vi "Camera Begin.vi"() -> ()   [LabVIEW 2013]
uses:
  <vilib>/Rock Robotics/WPI/Camera/WPI_CameraWhite Balance Values.ctl
  <vilib>/Rock Robotics/WPI/Camera/WPI_CameraFrameRate.ctl
  <vilib>/Rock Robotics/WPI/Camera/WPI_CameraExposure Values.ctl
  <vilib>/Rock Robotics/WPI/Camera/WPI_CameraImageSize.ctl
  <vilib>/Rock Robotics/SystemInterfaces/AI/FPGA_AIChannel.ctl
  <vilib>/Rock Robotics/SystemInterfaces/Typedef/FPGA_TypedefAnalogModule.ctl
panel:
  in  "Camera 2":T5={"Camera Address"="192.168.0.90", "Compression"=0, "White Balance"=enum."Auto", "Frame Rate (fps)"=30, "Exposure"=enum."Auto", "Image Size"=enum."320x240", "Brightness"=50, "refnum name"="My Camera RefNum"} {"Brightness" min=0 max=100; "Frame Rate (fps)" min=1 max=30; "Compression" min=0 max=100}
  in  "Camera 1":T5={"Camera Address"="192.168.0.90", "Compression"=0, "White Balance"=enum."Auto", "Frame Rate (fps)"=30, "Exposure"=enum."Auto", "Image Size"=enum."320x240", "Brightness"=50, "refnum name"="My Camera RefNum"} {"Brightness" min=0 max=100; "Frame Rate (fps)" min=1 max=30; "Compression" min=0 max=100}
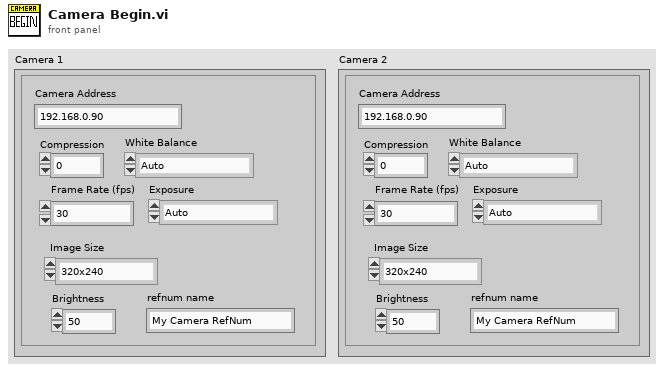
[diagram p1: front panel]
types:
  T1 = typedef "WPI_CameraWhite Balance Values.ctl" = enum16{"Auto", "Fixed indoor", "Fixed outdoor 1", "Fixed outdoor 2", "Fixed fluorescent 1", "Fixed fluorescent 2", "Hold current"}
  T2 = typedef "WPI_CameraFrameRate.ctl" = u32
  T3 = typedef "WPI_CameraExposure Values.ctl" = enum16{"Auto", "Flicker-free 50 Hz", "Flicker-free 60 Hz", "Hold current"}
  T4 = typedef "WPI_CameraImageSize.ctl" = enum16{"640x480", "320x240", "160x120"}
  T5 = cluster{"Camera Address":string, "Compression":i32, "White Balance":T1, "Frame Rate (fps)":T2, "Exposure":T3, "Image Size":T4, "Brightness":i32, "refnum name":string}
  T6 = typedef "FPGA_TypedefAnalogModule.ctl" = enum16{"Analog Module 1", "Analog Module 2"}
  T7 = typedef "FPGA_AIChannel.ctl" = enum8{"AI 1", "AI 2", "AI 3", "AI 4", "AI 5", "AI 6", "AI 7", "AI 8", "Invalid"}
  T8 = typedef "WPI_AnalogChannelDevRef.ctl" = cluster{"DevStatus":errorcluster, "Analog Module":T6, "Analog Channel":T7}
  T9 = typedef "WPI_CameraDevRef.ctl" = cluster{"Camera Address":string, "CameraStatus":errorcluster, "Acquire Image Notifier":refnum<notifier>}
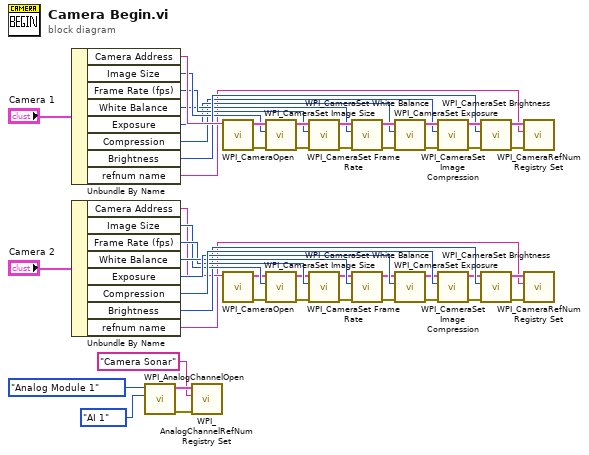
[diagram p0: block diagram]
diagram:
  n1 = Unbundle By Name("Camera 1") -> ("Camera Address"=w36:string, "Image Size"=w34:T4, "Frame Rate (fps)"=w33:T2, "White Balance"=w32:T1, "Exposure"=w31:T3, "Compression"=w30:i32, "Brightness"=w35:i32, "refnum name"=w7:string)
  n2 = Unbundle By Name("Camera 2") -> ("Camera Address"=w23:string, "Image Size"=w25:T4, "Frame Rate (fps)"=w26:T2, "White Balance"=w27:T1, "Exposure"=w28:T3, "Compression"=w29:i32, "Brightness"=w24:i32, "refnum name"=w6:string)
  n3 = call <vilib>:"WPI_AnalogChannelOpen.vi"("Analog Channel"=FPGA_AIChannel."AI 1", "Analog Module (Module 1)"=FPGA_TypedefAnalogModule."Analog Module 1") -> ("error out"=w4:errorcluster, "AIDeviceRef"=w5:T8)  [unwired: 8 in]
  n4 = call <vilib>:"WPI_AnalogChannelRefNum Registry Set.vi"("error in (no error)"=w4, "refnum name"="Camera Sonar", "AIDeviceRef"=w5) -> ()  [unwired: 7 in, 2 out]
  n5 = call <vilib>:"WPI_CameraOpen.vi"("Camera Address"=w36) -> ("error out"=w45:errorcluster, "CameraDevRef"=w46:T9)  [unwired: 1 in, 8 out]
  n6 = call <vilib>:"WPI_CameraOpen.vi"("Camera Address"=w23) -> ("error out"=w14:errorcluster, "CameraDevRef"=w13:T9)  [unwired: 1 in, 8 out]
  n7 = call <vilib>:"WPI_CameraSet Image Size.vi"("error in (no error)"=w45, "Image Size"=w34, "CameraDevRef"=w46) -> ("error out"=w44:errorcluster, "CameraDevRef Out"=w47:T9)  [unwired: 7 out]
  n8 = call <vilib>:"WPI_CameraSet Image Size.vi"("error in (no error)"=w14, "Image Size"=w25, "CameraDevRef"=w13) -> ("error out"=w15:errorcluster, "CameraDevRef Out"=w12:T9)  [unwired: 7 out]
  n9 = call <vilib>:"WPI_CameraSet Frame Rate.vi"("error in (no error)"=w44, "Frame Rate (fps)"=w33, "CameraDevRef"=w47) -> ("error out"=w43:errorcluster, "CameraDevRef Out"=w49:T9)  [unwired: 7 out]
  n10 = call <vilib>:"WPI_CameraSet Frame Rate.vi"("error in (no error)"=w15, "Frame Rate (fps)"=w26, "CameraDevRef"=w12) -> ("error out"=w16:errorcluster, "CameraDevRef Out"=w10:T9)  [unwired: 7 out]
  n11 = call <vilib>:"WPI_CameraSet White Balance.vi"("error in (no error)"=w43, "White Balance"=w32, "CameraDevRef"=w49) -> ("error out"=w42:errorcluster, "CameraDevRef Out"=w48:T9)  [unwired: 7 out]
  n12 = call <vilib>:"WPI_CameraSet White Balance.vi"("error in (no error)"=w16, "White Balance"=w27, "CameraDevRef"=w10) -> ("error out"=w17:errorcluster, "CameraDevRef Out"=w11:T9)  [unwired: 7 out]
  n13 = call <vilib>:"WPI_CameraSet Exposure.vi"("error in (no error)"=w42, "Exposure"=w31, "CameraDevRef"=w48) -> ("error out"=w41:errorcluster, "CameraDevRef Out"=w51:T9)  [unwired: 7 out]
  n14 = call <vilib>:"WPI_CameraSet Exposure.vi"("error in (no error)"=w17, "Exposure"=w28, "CameraDevRef"=w11) -> ("error out"=w18:errorcluster, "CameraDevRef Out"=w8:T9)  [unwired: 7 out]
  n15 = call <vilib>:"WPI_CameraSet Image Compression.vi"("error in (no error)"=w41, "Compression"=w30, "CameraDevRef"=w51) -> ("error out"=w40:errorcluster, "CameraDevRef Out"=w50:T9)  [unwired: 7 out]
  n16 = call <vilib>:"WPI_CameraSet Image Compression.vi"("error in (no error)"=w18, "Compression"=w29, "CameraDevRef"=w8) -> ("error out"=w19:errorcluster, "CameraDevRef Out"=w9:T9)  [unwired: 7 out]
  n17 = call <vilib>:"WPI_CameraSet Brightness.vi"("error in (no error)"=w40, "Brightness"=w35, "CameraDevRef"=w50) -> ("error out"=w38:errorcluster, "CameraDevRef Out"=w39:T9)  [unwired: 7 out]
  n18 = call <vilib>:"WPI_CameraSet Brightness.vi"("error in (no error)"=w19, "Brightness"=w24, "CameraDevRef"=w9) -> ("error out"=w21:errorcluster, "CameraDevRef Out"=w20:T9)  [unwired: 7 out]
  n19 = call <vilib>:"WPI_CameraRefNum Registry Set.vi"("error in (no error)"=w38, "refnum name"=w7, "CameraDevRef"=w39) -> ()  [unwired: 9 out]
  n20 = call <vilib>:"WPI_CameraRefNum Registry Set.vi"("error in (no error)"=w21, "refnum name"=w6, "CameraDevRef"=w20) -> ()  [unwired: 9 out]
